vi "Find All IO Variables.vi"(8 "error in":errorcluster, 10 "Path":path) -> (0 "error out":errorcluster, 2 "Tags":T1[](array[typedef]))   [LabVIEW 2013, in "Scan Engine editor node.lvclass"]
uses:
  Scan Engine editor node.lvclass
  configuration/Line.ctl
  <vilib>/NI/Tag Bus Module Framework/channel/TBM channel.lvclass
  <vilib>/NI/Tag Bus Module Framework/channel/channel classification.ctl
  <vilib>/NI/Tag Bus/tag/Data Type.ctl
  <vilib>/Utility/VariantDataType/VariantType.lvlib
  <vilib>/NI/Tag Bus/tag/tag descriptor.lvclass
  configuration/Scan Engine configuration.lvclass
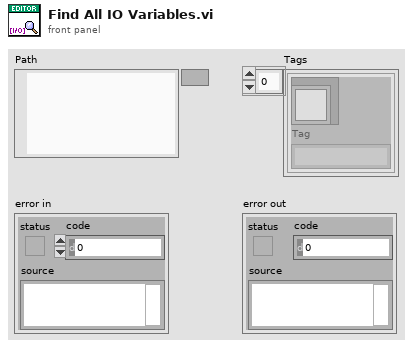
[diagram p1: front panel]
types:
  T1 = typedef "Scan Engine configuration.lvclass/Line.ctl" = cluster{"channel":refnum<class "TBM channel.lvclass">, "Tag":string}
  T2 = typedef "tag bus.lvlib/tag descriptor.lvclass/Data Type.ctl" = enum16{"Double", "Single", "I64", "I32", "I16", "I8", "U64", "U32", "U16", "U8", "Boolean", "String", "Array of Double", "Array of Single", "Array of I64", "Array of I32", "Array of I16", "Array of I8", "Array of U64", "Array of U32", "Array of U16", "Array of U8", "Array of Boolean", "Array of String"}
  T3 = typedef "TBM channel.lvclass/channel classification.ctl" = enum16{"input data", "output data", "processing parameter", "processing result"}
  T4 = typedef "VariantType.lvlib/Type.ctl" = enum8{"Invalid Type", "Void", "I8", "I16", "I32", "I64", "U8", "U16", "U32", "U64", "Single Float", "Double Float", "Extended Float", "Single Complex", "Double Complex", "Extended Complex", "Enum U8", "Enum U16", "Enum U32", "Enum U64", "Single Float With Unit", "Double Float With Unit", "Extended Float With Unit", "Single Complex with Unit", "Double Complex with Unit", "Extended Complex with Unit", "Boolean", "String", "Path", "Picture", "Tag", "Array", "Cluster", "Variant", "LV Variant", "Waveform", "Timestamp", "Digital Waveform", "Digital Data", "ExpressData", "Refnum", "External Data", "VI", "Poly VI", "LabVIEW Class Instance", "Fixed Point"}
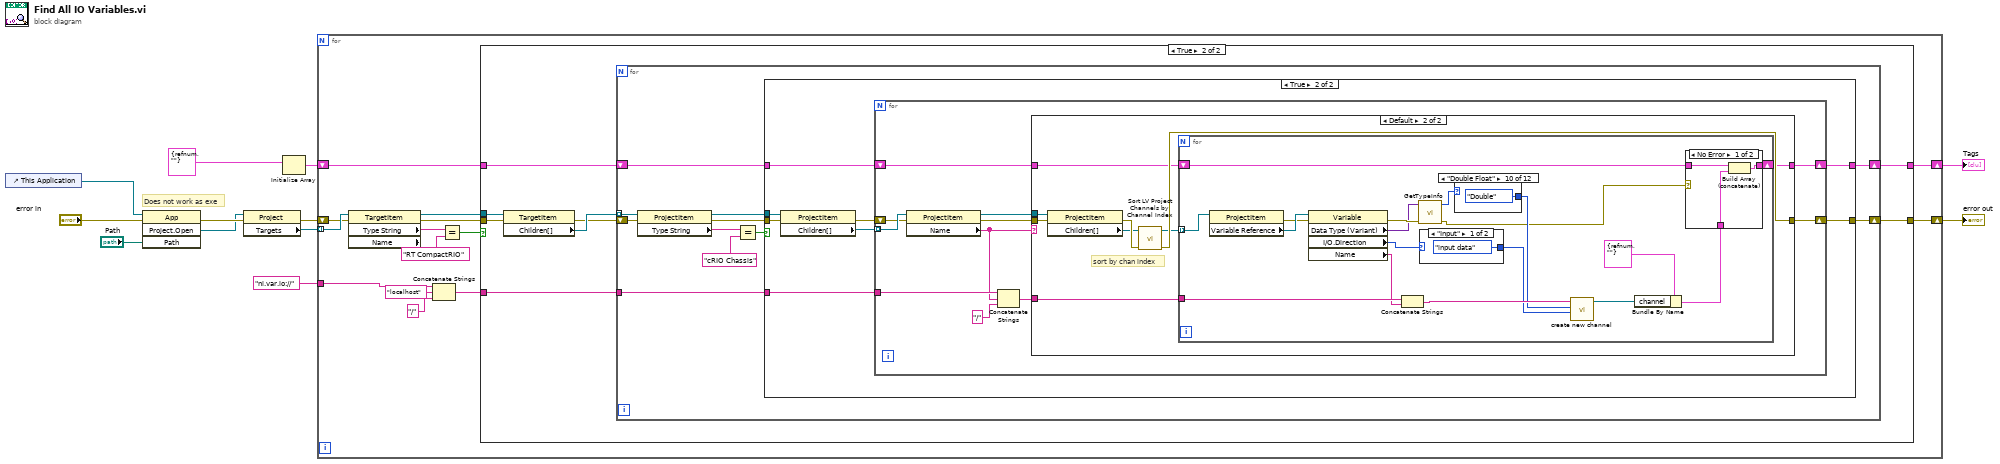
[diagram p0: block diagram]
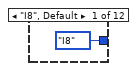
[diagram p6: hidden frame]
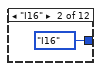
[diagram p7: hidden frame]
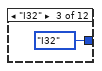
[diagram p8: hidden frame]
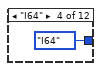
[diagram p9: hidden frame]
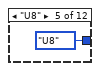
[diagram p10: hidden frame]
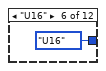
[diagram p11: hidden frame]
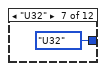
[diagram p12: hidden frame]
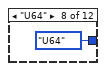
[diagram p13: hidden frame]
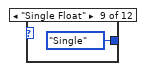
[diagram p14: hidden frame]
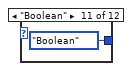
[diagram p15: hidden frame]
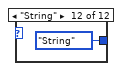
[diagram p16: hidden frame]
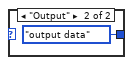
[diagram p17: hidden frame]
diagram:
  # "Does not work as exe"
  n1 = control-ref of="This Application"() -> (w5:refnum<vi>)
  n2 = invoke class="App" method="Project.Open"(reference=w5, error in="error in", "Path"="Path") -> (error out=w7:errorcluster, "Project:Open"=w6:refnum<vi>)  [unwired: 1 in, 2 out]
  n3 = property class="Project"(reference=w6, error in=w7) -> (error out=w9:errorcluster, "Targets"=w8:refnum<vi>[])  [unwired: 1 out]
  n4 = Initialize Array(T1 {"channel"=refnum, "Tag"=""} ("Line")) -> (w3:T1[])  [unwired: 1 in]
  n5 = for {
    tunnel: w8 -> [w26] mode=indexing
    shift-right: [w19] -> w10
    shift-left: w9 -> [w21]
    shift-right: [w18] -> w4
    shift-left: w3 -> [w17]
    tunnel: "ni.var.io://" -> [w14]
    n6 = property class="TargetItem" props=["Type String", "Name"](reference=w26, error in=w21) -> (reference out=w22:refnum<vi>, error out=w20:errorcluster, "Type String"=w25:string)  [unwired: 1 out]
    n7 = Concatenate Strings(w14, "localhost" ("string"), "/" ("string")) -> (w15:string)
    n8 = Equal?(x=w25, y="RT CompactRIO" ("Type String")) -> (x = y?=w23:bool)
    n9 = case shown="True" w23 {
      tunnel: w22 -> [_ w33]
      tunnel: w20 -> [w28 w32]
      tunnel: [w28 w34] -> w19
      tunnel: [w27 w30] -> w18
      tunnel: w17 -> [w27 w31]
      tunnel: w15 -> [_ w29]
      frame False {
      }
      frame True {
        n10 = property class="TargetItem"(reference=w33, error in=w32) -> (error out=w35:errorcluster, "Children[]"=w36:refnum<vi>[])  [unwired: 1 out]
        n11 = for {
          tunnel: w36 -> [w47] mode=indexing
          shift-right: [w40] -> w34
          shift-left: w35 -> [w42]
          shift-right: [w38] -> w30
          shift-left: w31 -> [w39]
          tunnel: w29 -> [w37]
          n12 = property class="ProjectItem"(reference=w47, error in=w42) -> (reference out=w43:refnum<vi>, error out=w41:errorcluster, "Type String"=w46:string)
          n13 = Equal?(x=w46, y="cRIO Chassis") -> (x = y?=w44:bool)
          n14 = case shown="True" w44 {
            tunnel: w43 -> [_ w57]
            tunnel: w41 -> [w49 w56]
            tunnel: [w49 w54] -> w40
            tunnel: w39 -> [w48 w52]
            tunnel: [w48 w51] -> w38
            tunnel: w37 -> [_ w50]
            frame False {
            }
            frame True {
              n15 = property class="ProjectItem"(reference=w57, error in=w56) -> (error out=w55:errorcluster, "Children[]"=w53:refnum<vi>[])  [unwired: 1 out]
              n16 = for {
                tunnel: w53 -> [w68] mode=indexing
                shift-right: [w64] -> w54
                shift-left: w55 -> [w65]
                shift-right: [w62] -> w51
                shift-left: w52 -> [w63]
                tunnel: w50 -> [w60]
                n17 = property class="ProjectItem"(reference=w68, error in=w65) -> (reference out=w67:refnum<vi>, error out=w66:errorcluster, "Name"=w59:string)
                n18 = Concatenate Strings(w60, w59, "/" ("string")) -> (w58:string)
                n19 = case shown="Default" w59 {
                  tunnel: w67 -> [_ w77]
                  tunnel: w66 -> [w70 w76]
                  tunnel: [w70 w78] -> w64
                  tunnel: w63 -> [w69 w75]
                  tunnel: [w69 w74] -> w62
                  tunnel: w58 -> [_ w73]
                  frame "FPGA Target" {
                  }
                  frame Default {
                    # "sort by chan index"
                    n20 = property class="ProjectItem"(reference=w77, error in=w76) -> (error out=w79:errorcluster, "Children[]"=w72:refnum<vi>[])  [unwired: 1 out]
                    n21 = call "Sort LV Project Channels by Channel Index.vi"("error in (no error)"=w79, "Project Channels in"=w72) -> ("error out"=w78:errorcluster, "Project Channels out"=w71:refnum<vi>[])  [unwired: 8 in]
                    n22 = for {
                      tunnel: w71 -> [w97] mode=indexing
                      shift-right: [w91] -> w74
                      shift-left: w75 -> [w92]
                      tunnel: w73 -> [w87]
                      n23 = property class="ProjectItem"(reference=w97) -> (error out=w94:errorcluster, "Variable Reference"=w96:refnum<vi>)  [unwired: 1 in, 1 out]
                      n24 = property class="Variable"(reference=w96, error in=w94) -> (error out=w95:errorcluster, "Data Type (Variant)"=w88:variant, "I/O.Direction"=w89:enum8{"Input", "Output"}, "Name"=w86:string)  [unwired: 1 out]
                      n25 = Concatenate Strings(w87, w86) -> (w85:string)
                      n26 = call <vilib>:"GetTypeInfo.vi"("error in (no error)"=w95, "Variant"=w88) -> ("error out"=w81:errorcluster, "Type Enum"=w93:T4)  [unwired: 5 in, 3 out]
                      n27 = case shown="\"Input\"" w89 {
                        tunnel: [channel_classification."input data" ("channel classification") channel_classification."output data" ("channel classification")] -> w84
                        frame "Input" {
                        }
                        frame "Output" {
                        }
                      }
                      n28 = case shown="\"Double Float\"" w93 {
                        tunnel: [Data_Type."I8" ("data type") Data_Type."I16" ("data type") Data_Type."I32" ("data type") Data_Type."I64" ("data type") Data_Type."U8" ("data type") Data_Type."U16" ("data type") Data_Type."U32" ("data type") Data_Type."U64" ("data type") Data_Type."Single" ("data type") Data_Type."Double" ("data type") Data_Type."Boolean" ("data type") Data_Type."String" ("data type")] -> w83
                        frame "I8", Default {
                        }
                        frame "I16" {
                        }
                        frame "I32" {
                        }
                        frame "I64" {
                        }
                        frame "U8" {
                        }
                        frame "U16" {
                        }
                        frame "U32" {
                        }
                        frame "U64" {
                        }
                        frame "Single Float" {
                        }
                        frame "Double Float" {
                        }
                        frame "Boolean" {
                        }
                        frame "String" {
                        }
                      }
                      n29 = call <vilib>:"create new channel.vi"("channel classification"=w84, "data type"=w83, "channel name"=w85) -> ("channel"=w82:refnum<class "TBM channel.lvclass">)  [unwired: 8 in]
                      n30 = Bundle By Name(cluster=T1 {"channel"=refnum, "Tag"=""} ("Line"), "channel"=w82) -> (w90:T1)
                      n31 = case shown="No Error" w81 {
                        tunnel: w92 -> [w100 w101]
                        tunnel: [w99 w101] -> w91
                        tunnel: w90 -> [w98 _]
                        frame No Error {
                          n32 = Build Array (concatenate)(w100, w98) -> (w99:T1[])
                        }
                        frame Error {
                        }
                      }
                    }
                  }
                }
              }
            }
          }
        }
      }
    }
  }
  "Tags" <- w4
  "error out" <- w10
